vi "SweepTresholdControl.vi"() -> ()   [LabVIEW 2009]
uses:
  <vilib>/Utility/NIReport.llb/NI_report.lvclass
  <vilib>/Utility/NIReport.llb/HTML/NI_HTML.lvclass
panel:
  out "Thresold":dbl
  in  "Channel":i8
  in  "Instrument VISA in":T1={"AWG VISA"="generadorpulsos", "Oscilloscope  VISA "="Oscilloscope", "Integration Board IP"="172.16.7.43", "connection ID"=refnum, "report out"=refnum, "report file path"=path "C:/Documents and Settings/CTA_LAB01/Desktop/L0_Asic/L0 Asic Test Data"}
  in  "Amp Scaler":dbl(slide)=1.110204081632653 scale=0.1..10.0
  in  "Voltage Input":dbl(slide)=0.21071428571428574 scale=0.05..0.8
  out "error out":errorcluster
  in  "error in":errorcluster
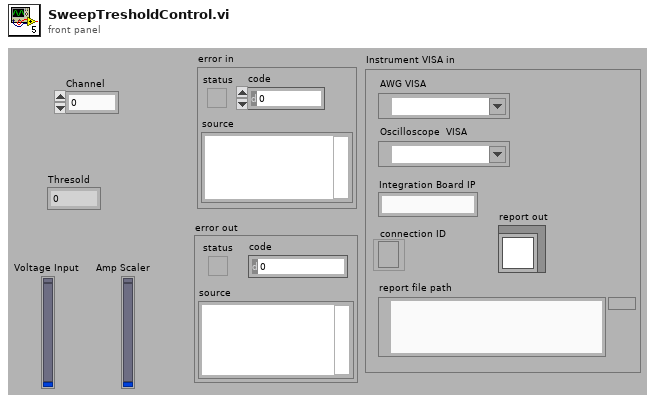
[diagram p1: front panel]
types:
  T1 = cluster{"AWG VISA":refnum<visa-resource-name>, "Oscilloscope  VISA ":refnum<visa-resource-name>, "Integration Board IP":string, "connection ID":refnum<k5>, "report out":refnum<class "NI_report.lvclass">, "report file path":path}
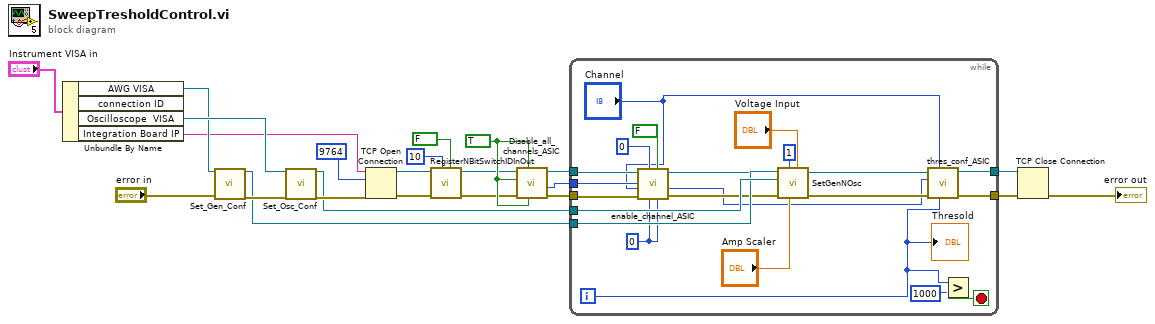
[diagram p0: block diagram]
diagram:
  w21 = TRUE ("Att_en_b")
  n1 = Unbundle By Name("Instrument VISA in") -> ("AWG VISA"=w10:refnum<visa-resource-name>, "Oscilloscope  VISA"=w11:refnum<visa-resource-name>, "Integration Board IP"=w6:string)  [unwired: 1 out]
  n2 = call "Set_Gen_Conf.vi"("AWG VISA"=w10, "error in (no error)"="error in") -> ("VISA resource name out"=w4:refnum<visa-resource-name>, "error out"=w8:errorcluster)  [unwired: 10 in, 6 out]
  n3 = call "Set_Osc_Conf.vi"("VISA resource name"=w11, "error in (no error)"=w8) -> ("VISA resource name out"=w5:refnum<visa-resource-name>, "error out"=w7:errorcluster)  [unwired: 16 in]
  n4 = TCP Open Connection(address=w6, remote port or service name=u16 9764, error in (no error)=w7) -> (connection ID=w16:refnum<k5>, error out=w18:errorcluster)  [unwired: 2 in]
  n5 = call "RegisterNBitSwitchIDInOut.vi"("Switch Bit"=FALSE ("maj/sum"), "N Bit"=u32 10 ("Att gain"), "error in (no error)"=w18, "connection ID"=w16) -> ("error out"=w17:errorcluster, "connection ID out"=w15:refnum<k5>)  [unwired: 5 in]
  n6 = call "Disable_all_channels_ASIC.vi"("CompBuf_en_b"=w21, "Att_en_b"=w21, "error in"=w17, "Clip_en_b"=w21, "connection ID"=w15) -> ("error out"=w1:errorcluster, "id_out"=w2:i32, "connection ID out"=w3:refnum<k5>)  [unwired: 4 in]
  n7 = while {
    tunnel: [w44] -> w20
    tunnel: [w43] -> w19
    tunnel: w1 -> [w33]
    tunnel: w2 -> [w28]
    tunnel: w3 -> [w31]
    tunnel: w5 -> [w39]
    tunnel: w4 -> [w38]
    i -> [w25]
    stop <- w26 stop-if-true
    w36 = u32 0 ("Ib_clipVb")
    n8 = call "enable_channel_ASIC.vi"("Clip_sel_b"=w36, "maj/sum"=FALSE, "Ib_clipVb"=w36, "Att gain"=u32 0, "error in"=w33, "Channel"="Channel", "id_in"=w28, "connection ID"=w31) -> ("error out"=w32:errorcluster, "id_out"=w29:i32, "connection ID out"=w30:refnum<k5>)  [unwired: 1 in]
    n9 = call "SetGenNOsc.vi"("Input Voltage"="Voltage Input", "Amp Scaler"="Amp Scaler", "NChannels"=1, "error in (no error)"=w32, "VISA resource name"=w39, "AWG VISA"=w38) -> ("error out 2"=w37:errorcluster)  [unwired: 5 in]
    n10 = call "thres_conf_ASIC.vi"("threshold"=w25, "Ring"="Channel", "error out 3"=w37, "Id in"=w29, "connection ID"=w30) -> ("error out 2"=w44:errorcluster, "connection ID out"=w43:refnum<k5>)  [unwired: 3 in, 2 out]
    n11 = Greater?(x=w25, y=u32 1000 ("Ib_clipVb")) -> (0:w26:bool)
    "Thresold" <- w25
  }
  n12 = TCP Close Connection(connection ID=w19, error in (no error)=w20) -> (error out=→"error out":errorcluster)  [unwired: 1 in, 1 out]
